vi "get channels removed since last load.vi"(8 "error in":errorcluster, 11 "fixed channel configuration in":refnum<class "fixed channel configuration.lvclass">) -> (0 "error out":errorcluster, 2 "removed":refnum<class "TBM channel.lvclass">[](array[class]), 3 "fixed channel configuration out":refnum<class "fixed channel configuration.lvclass">)   [LabVIEW 2013, in "fixed channel configuration.lvclass"]
uses:
  fixed channel configuration.lvclass
  <vilib>/NI/Tag Bus Module Framework/channel/TBM channel.lvclass
  fixed channel configuration.lvclass/fixed channel configuration.ctl
  <vilib>/NI/Tag Bus/tag/tag descriptor.lvclass/tag descriptor.ctl
  <vilib>/NI/Tag Bus Module Framework/channel/TBM channel.lvclass/TBM channel.ctl
  <vilib>/NI/Tag Bus/tag/read data type.vi
  <vilib>/NI/Tag Bus Module Framework/channel/Read channel classification.vi
  <vilib>/NI/Tag Bus/tag/read tag name.vi
  <vilib>/NI/Tag Bus/tag/tag descriptor.lvclass
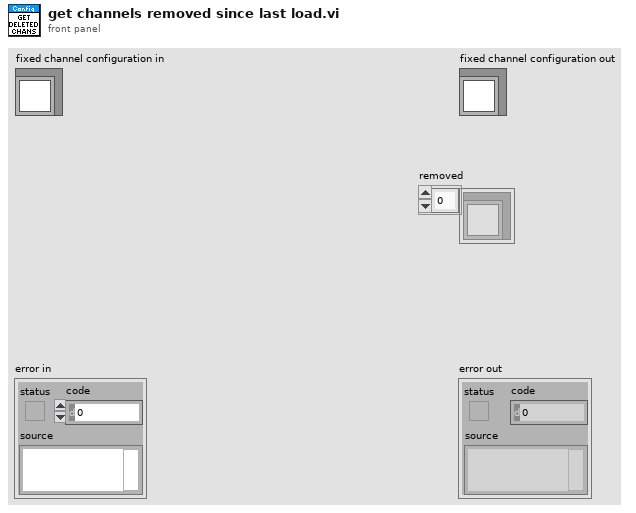
[diagram p1: front panel]
types:
  T1 = typedef "tag bus.lvlib/tag descriptor.lvclass/Data Type.ctl" = enum16{"Double", "Single", "I64", "I32", "I16", "I8", "U64", "U32", "U16", "U8", "Boolean", "String", "Array of Double", "Array of Single", "Array of I64", "Array of I32", "Array of I16", "Array of I8", "Array of U64", "Array of U32", "Array of U16", "Array of U8", "Array of Boolean", "Array of String"}
  T2 = typedef "TBM channel.lvclass/channel classification.ctl" = enum16{"input data", "output data", "processing parameter", "processing result"}
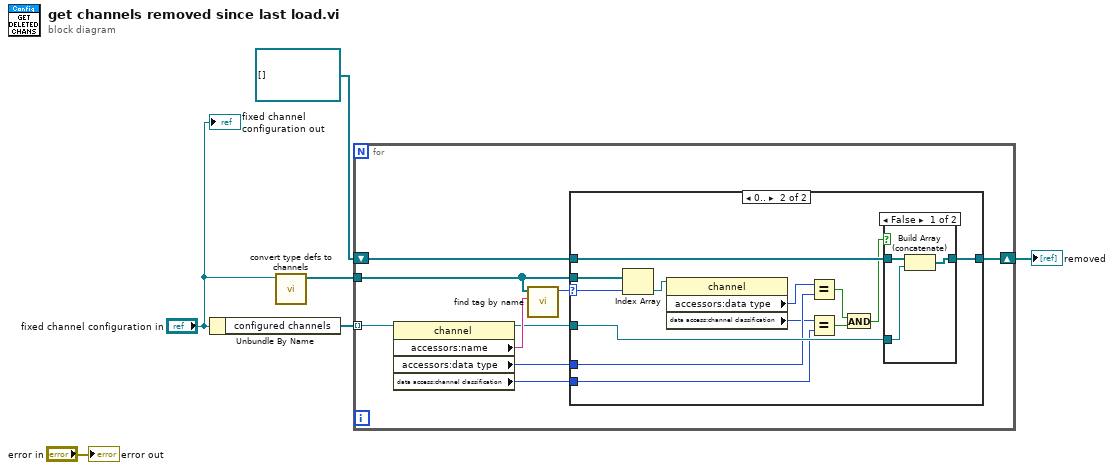
[diagram p0: block diagram]
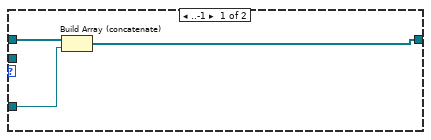
[diagram p2: hidden frame]
diagram:
  n1 = Unbundle By Name("fixed channel configuration in") -> ("configured channels"=w5:refnum<class "TBM channel.lvclass">[])
  n2 = call "convert type defs to channels.vi"("fixed channel configuration"="fixed channel configuration in") -> ("Array out"=w6:refnum<class "TBM channel.lvclass">[])  [unwired: 9 in, 1 out]
  n3 = for {
    tunnel: w5 -> [w15] mode=indexing
    shift-right: [w9] -> w1
    shift-left: refnum<class "TBM channel.lvclass">[] [] ("Array out") -> [w10]
    tunnel: w6 -> [w8]
    n4 = property class="channel"(reference=w15) -> (reference out=w11:refnum<class "TBM channel.lvclass">, "accessors:name"=w14:string, "accessors:data type"=w12:T1, "data access:channel classification"=w7:T2)  [unwired: 1 in, 1 out]
    n5 = call <vilib>:"find tag by name.vi"("name"=w14, "tags in"=w8) -> ("index"=w13:i32)  [unwired: 9 in]
    n6 = case shown="0.." w13 {
      selector: w13 -> [_ w30]
      tunnel: w12 -> [_ w24]
      tunnel: w11 -> [w17 w26]
      tunnel: w10 -> [w18 w28]
      tunnel: [w16 w27] -> w9
      tunnel: w8 -> [_ w31]
      tunnel: w7 -> [_ w19]
      frame ..-1 {
        n7 = Build Array (concatenate)(w18, w17) -> (w16:refnum<class "TBM channel.lvclass">[])
      }
      frame 0.. {
        n8 = Index Array(array=w31, index=w30) -> (element=w29:refnum<class "TBM channel.lvclass">)
        n9 = property class="channel"(reference=w29) -> ("accessors:data type"=w25:T1, "data access:channel classification"=w20:T2)  [unwired: 1 in, 2 out]
        n10 = Equal?(x=w25, y=w24) -> (x = y?=w23:bool)
        n11 = Equal?(x=w20, y=w19) -> (x = y?=w21:bool)
        n12 = And(x=w23, y=w21) -> (x .and. y?=w22:bool)
        n13 = case shown="False" w22 {
          tunnel: w28 -> [w34 w35]
          tunnel: [w33 w35] -> w27
          tunnel: w26 -> [w32 _]
          frame False {
            n14 = Build Array (concatenate)(w34, w32) -> (w33:refnum<class "TBM channel.lvclass">[])
          }
          frame True {
          }
        }
      }
    }
  }
  "removed" <- w1
  "error out" <- "error in"
  "fixed channel configuration out" <- "fixed channel configuration in"
